vi "单个流程写入.vi"(5 "简易流程Id":u16, 6 "是否是简易流程":bool, 7 "添加的路径":path, 8 "error in (no error)":errorcluster caption="错误输入（无错误）", 9 "量程":enum16{"低量程", "高量程"}(ring), 10 "测量模式":T1(ring), 11 "测量参数":u16(ring) items=["总氮"=2, "总磷"=1, "氨氮"=3, "COD"=22]) -> (0 "error out":errorcluster caption="错误输出", 3 "大小":i32)   [LabVIEW 2022 SP3, in "斯坦道总氮.lvlib"]
uses:
  <vilib>/Plasmionique/MB Master/MB Master.lvlib
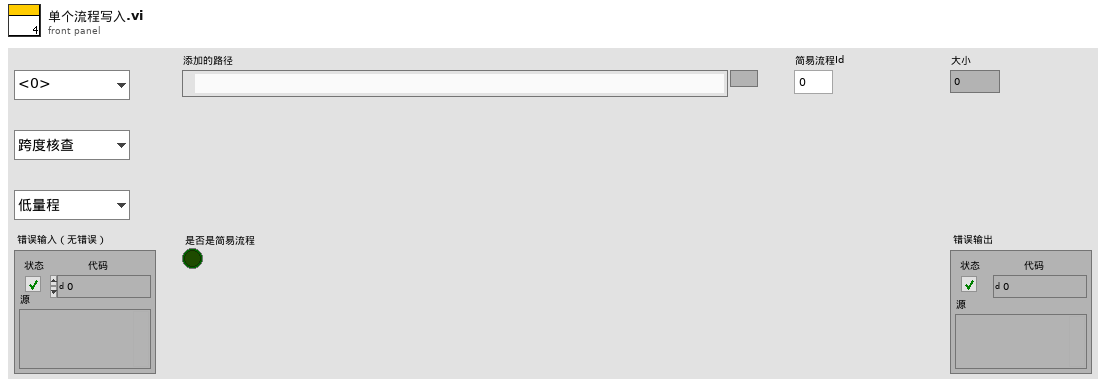
[diagram p1: front panel]
types:
  T1 = enum16{"跨度核查", "水样测量", "零点核查", "标样核查", "加标回收", "平行样测试", "空白校准", "标样校准", "空白测试"}
  T2 = cluster{"测量参数":u16, "测量模式":enum16{"跨度核查", "水样测量", "零点核查", "标样核查", "加标回收", "平行样测试", "空白校准", "标样校准", "空白测试"}, "量程":enum16{"低量程", "高量程"}}
  T3 = typedef "SingleStepTestV3.lvlib/SingleStepTestV3.lvclass/仪器版本.ctl" = enum16{"V3.1版", "V4版", "V3版", "V4.2版"}
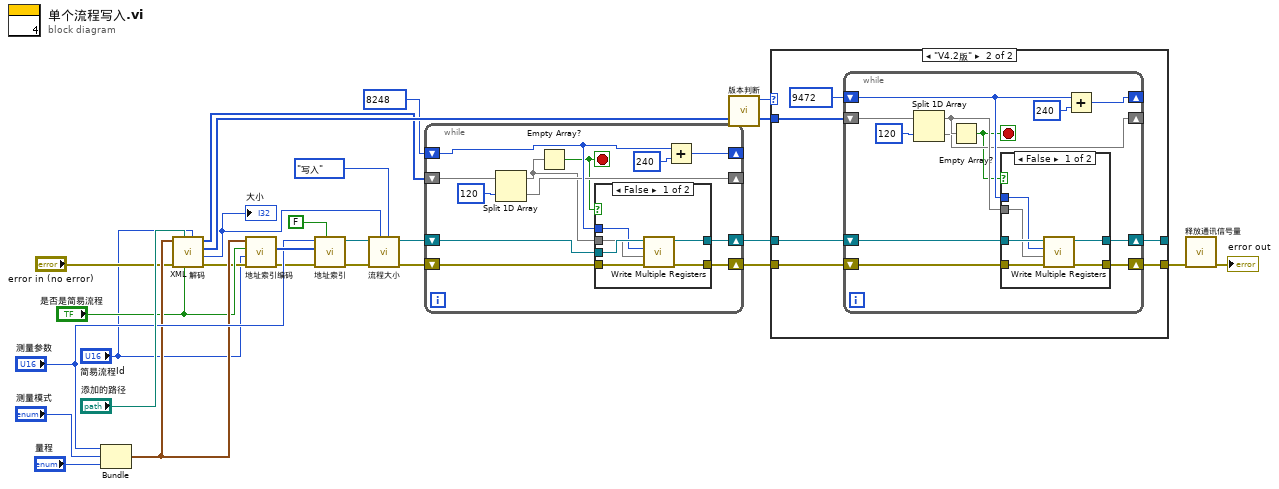
[diagram p0: block diagram]
diagram:
  n1 = Bundle("测量参数"="测量参数", "测量模式"="测量模式", "量程"="量程") -> (w6:T2)  [unwired: 1 in]
  n2 = call "XML 解码.vi"("简易流程Id"="简易流程Id", "是否是简易流程"="是否是简易流程", "添加的路径"="添加的路径", "error in (no error)"="error in (no error)", "参数簇"=w6) -> ("error out"=w3:errorcluster, "大小"=w18:i32, "步骤文本"=w19:u16[], "步骤详情"=w14:u16[])  [unwired: 3 in]
  "大小" <- w18
  n3 = call "地址索引编码.vi"("error in (no error)"=w3, "简易流程Id"="简易流程Id", "是否是简易流程"="是否是简易流程", "参数簇"=w6) -> ("error out"=w2:errorcluster, "数组"=w16:u16[])  [unwired: 6 in]
  n4 = call "地址索引.vi"("4.2写公式？"=FALSE ("写流程？"), "error in (no error)"=w2, "values"=w16, "测量参数"="测量参数") -> ("error out"=w26:errorcluster, "MB session out"=w25:refnum<class "MB_Master.lvclass">)  [unwired: 6 in]
  n5 = call "流程大小.vi"("功能"=enum16{"写入", "读取"}."写入", "大小"=w18, "error in (no error)"=w26, "MB session in"=w25) -> ("error out"=w10:errorcluster, "MB session out"=w15:refnum<class "MB_Master.lvclass">)  [unwired: 5 in, 1 out]
  n6 = while {
    shift-right: [w36] -> w12
    shift-left: w15 -> [w37]
    shift-right: [w30] -> _
    shift-left: w14 -> [w38]
    shift-right: [w35] -> w11
    shift-left: w10 -> [w34]
    shift-right: [w32] -> _
    shift-left: u16 8248 ("starting address") -> [w31]
    stop <- w28 stop-if-true
    n7 = Split 1D Array(array=w38, index=120 ("索引")) -> (first subarray=w27:u16[], second subarray=w30:u16[])
    n8 = Empty Array?(array=w27) -> (empty?=w28:bool)
    n9 = case shown="False" w28 {
      tunnel: w37 -> [w44 w46]
      tunnel: w31 -> [w43 _]
      tunnel: [w42 w46] -> w36
      tunnel: w27 -> [w41 _]
      tunnel: [w40 w45] -> w35
      tunnel: w34 -> [w39 w45]
      frame False {
        n10 = call <vilib>:"Write Multiple Registers.vi"("error in (no error)"=w39, "values"=w41, "starting address"=w43, "MB session in"=w44) -> ("error out"=w40:errorcluster, "MB session out"=w42:refnum<class "MB_Master.lvclass">)  [unwired: 6 in]
      }
      frame True {
      }
    }
    n11 = Add(x=w31, y=u16 240) -> (x+y=w32:u16)
  }
  n12 = call "版本判断.vi"() -> ("仪器版本"=w20:T3)  [unwired: 11 in]
  n13 = case shown="\"V4.2版\"" w20 {
    tunnel: w12 -> [w48 w54]
    tunnel: w11 -> [w47 w52]
    tunnel: [w47 w51] -> w21
    tunnel: w19 -> [_ w50]
    tunnel: [w48 w49] -> _
    frame "V3.1版", Default {
    }
    frame "V4.2版" {
      n14 = while {
        shift-right: [w65] -> w49
        shift-left: w54 -> [w66]
        shift-right: [w60] -> _
        shift-left: u16 9472 ("starting address") -> [w59]
        shift-right: [w58] -> w51
        shift-left: w52 -> [w64]
        shift-right: [w56] -> _
        shift-left: w50 -> [w63]
        stop <- w55 stop-if-true
        n15 = Split 1D Array(array=w63, index=120 ("索引")) -> (first subarray=w57:u16[], second subarray=w56:u16[])
        n16 = Empty Array?(array=w57) -> (empty?=w55:bool)
        n17 = case shown="False" w55 {
          tunnel: w66 -> [w72 w74]
          tunnel: [w71 w74] -> w65
          tunnel: w64 -> [w70 w73]
          tunnel: w59 -> [w69 _]
          tunnel: [w68 w73] -> w58
          tunnel: w57 -> [w67 _]
          frame False {
            n18 = call <vilib>:"Write Multiple Registers.vi"("error in (no error)"=w70, "values"=w67, "starting address"=w69, "MB session in"=w72) -> ("error out"=w68:errorcluster, "MB session out"=w71:refnum<class "MB_Master.lvclass">)  [unwired: 6 in]
          }
          frame True {
          }
        }
        n19 = Add(x=w59, y=u16 240) -> (x+y=w60:u16)
      }
    }
  }
  n20 = call "释放通讯信号量.vi"("error in (no error)"=w21) -> ("error out"=→"error out":errorcluster)  [unwired: 10 in]
